vi "Write String Array Units.vi"(5 "Total_1":dbl, 7 "HHV_1":dbl, 8 "Error In":errorcluster, 9 "Gross Heating Value, Vol (Real, Dry)":dbl=1000.0 min=900.0 max=2600.0 step=1.0, 10 "Header Array":string[](array[string]), 11 "Data Cluster":T1) -> (0 "Error Out":errorcluster, 2 "Gas Rate (BTU/hr)":dbl, 3 "String Data":string[][](array[string]))   [LabVIEW 2020]
uses:
  Data Cluster.ctl
panel:
  in  "Header Array Debug":string[](array[string])=["Time Stamp", "Absolute Pressure", "Gauge/Diff. Pressure", "BarometricPressure", "Temperature", "Uncorrected", "Corrected", "Totalizer", "Tot. Timer", "Tot. Avg. Flow", "Tot. Peak Flow", "Gas Selected"]
  # "Totalizer Timer"
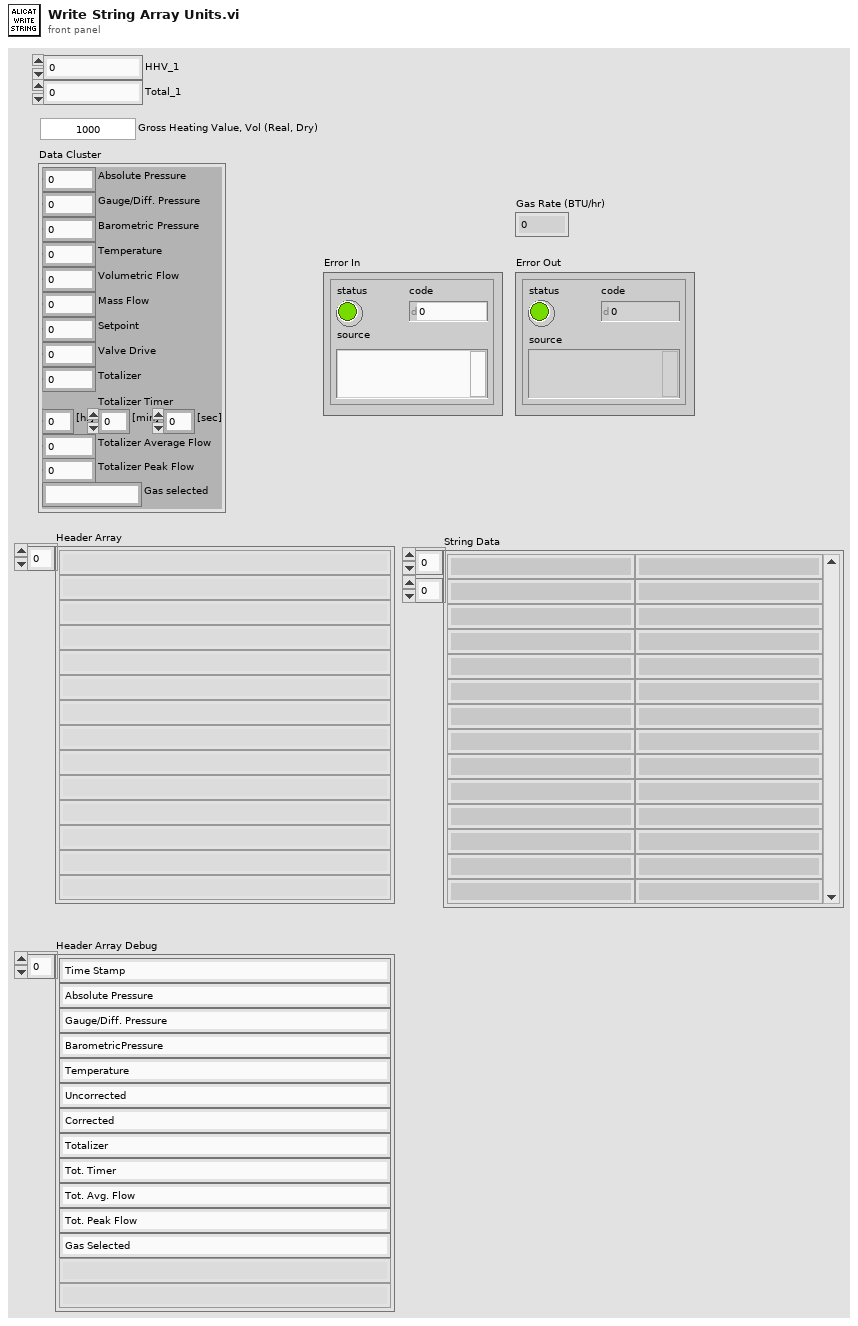
[diagram p1: front panel]
types:
  T1 = typedef "Data Cluster.ctl" = cluster{"Absolute Pressure":dbl, "Gauge/Diff. Pressure":dbl, "Barometric Pressure":dbl, "Temperature":dbl, "Volumetric Flow":dbl, "Mass Flow":dbl, "Setpoint":dbl, "Valve Drive":dbl, "Totalizer":dbl, "[hr]":dbl, "[min]":dbl, "[sec]":dbl, "Totalizer Average Flow":dbl, "Totalizer Peak Flow":dbl, "Gas selected":string}
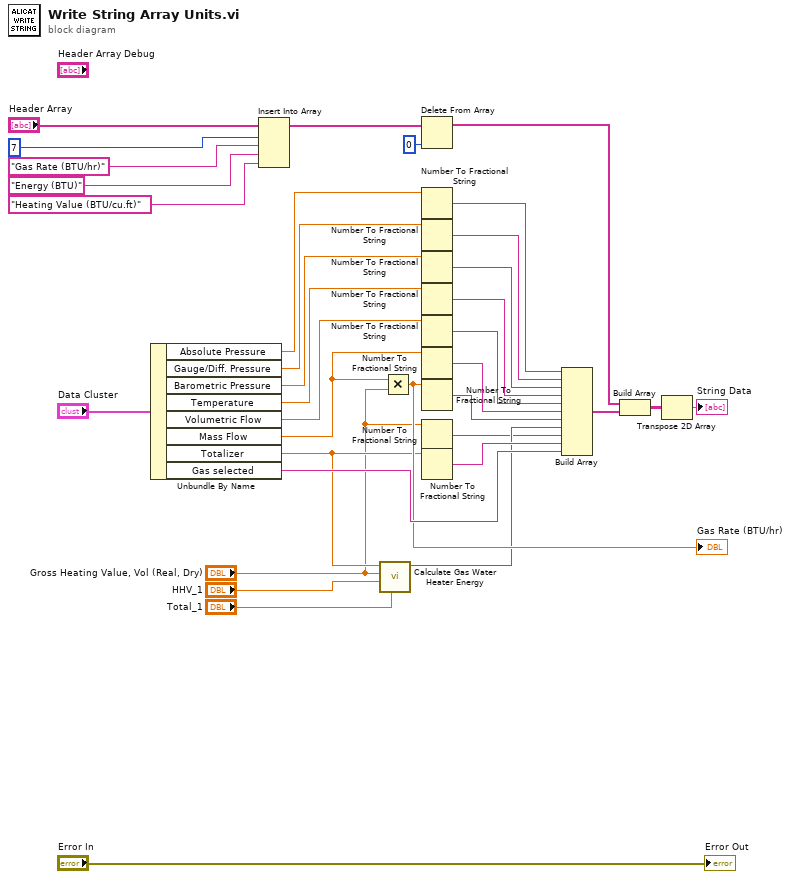
[diagram p0: block diagram]
diagram:
  n1 = Unbundle By Name("Data Cluster") -> ("Absolute Pressure"=w29:dbl, "Gauge/Diff. Pressure"=w30:dbl, "Barometric Pressure"=w31:dbl, "Temperature"=w32:dbl, "Volumetric Flow"=w33:dbl, "Mass Flow"=w17:dbl, "Totalizer"=w10:dbl, "Gas selected"=w21:string)
  n2 = Insert Into Array(array="Header Array", index=7, new element #1="Gas Rate (BTU/hr)" ("new element/subarray"), new element #2="Energy (BTU)" ("new element/subarray"), new element #3="Heating Value (BTU/cu.ft)" ("new element/subarray")) -> (w12:string[])
  n3 = call "Calculate Gas Water Heater Energy.vi"("Total_1"="Total_1", "HHV_1"="HHV_1", "Gross Heating Value, Vol (Real, Dry) in"="Gross Heating Value, Vol (Real, Dry)", "Totalizer"=w10) -> ("Total Energy"=w5:string)  [unwired: 4 in, 3 out]
  n4 = Multiply(x=w17, y="Gross Heating Value, Vol (Real, Dry)") -> (x*y=w16:dbl)
  "Gas Rate (BTU/hr)" <- w16
  n5 = Delete From Array(array=w12, index=0) -> (array with subset deleted=w4:string[])  [unwired: 1 in, 1 out]
  n6 = Number To Fractional String(number=w29) -> (F-format string=w27:string)  [unwired: 3 in]
  n7 = Number To Fractional String(number=w30) -> (F-format string=w26:string)  [unwired: 3 in]
  n8 = Number To Fractional String(number=w31) -> (F-format string=w25:string)  [unwired: 3 in]
  n9 = Number To Fractional String(number=w32) -> (F-format string=w24:string)  [unwired: 3 in]
  n10 = Number To Fractional String(number=w33) -> (F-format string=w23:string)  [unwired: 3 in]
  n11 = Number To Fractional String(number=w17) -> (F-format string=w22:string)  [unwired: 3 in]
  n12 = Number To Fractional String(number=w16) -> (F-format string=w15:string)  [unwired: 3 in]
  n13 = Number To Fractional String(number="Gross Heating Value, Vol (Real, Dry)") -> (F-format string=w1:string)  [unwired: 3 in]
  n14 = Number To Fractional String(number=w10) -> (F-format string=w11:string)  [unwired: 3 in]
  n15 = Build Array(w27, w26, w25, w24, w23, w22, w15, w5, w1, w11, w21) -> (w20:string[])
  n16 = Build Array(w4, w20) -> (w34:string[][])
  n17 = Transpose 2D Array(2D array=w34) -> (transposed array=→"String Data":string[][])
  "Error Out" <- "Error In"
